vi "wfm_feature set_search_plot_pos.vi"(8 "error in (no error)":errorcluster, 10 "new search plot pos":cluster{"Array":cluster{"X":dbl, "Y":dbl}[]}, 11 "wfm_feature in":refnum<class "wfm_feature.lvclass">) -> (0 "error out":errorcluster, 3 "wfm_feature out":refnum<class "wfm_feature.lvclass">)   [LabVIEW 2018, in "wfm_feature.lvclass"]
uses:
  wfm_feature.lvclass
  wfm_feature.lvclass/wfm_feature.ctl
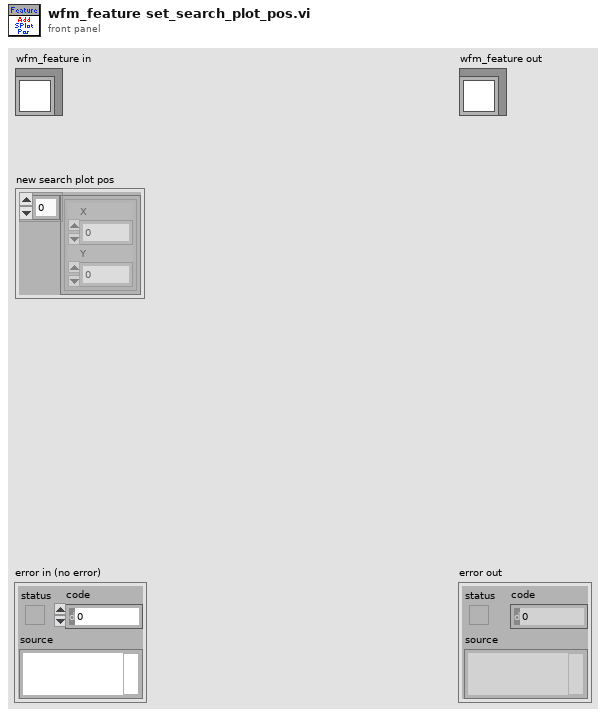
[diagram p1: front panel]
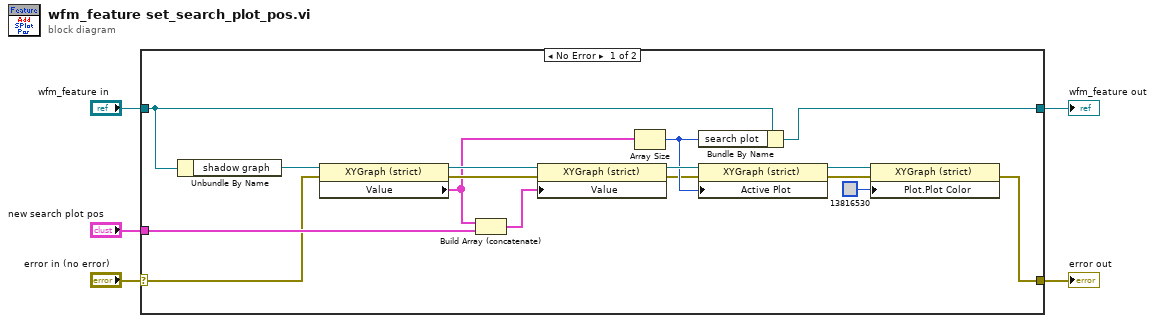
[diagram p0: block diagram]
diagram:
  n1 = case shown="No Error" "error in (no error)" {
    selector: "error in (no error)" -> [w14 w23]
    tunnel: [w6 w23] -> w4
    tunnel: [w15 w22] -> w2
    tunnel: "wfm_feature in" -> [w13 w22]
    tunnel: "new search plot pos" -> [w18 _]
    frame No Error {
      n2 = Unbundle By Name(w13) -> ("shadow graph"=w21:refnum<vi>)
      n3 = property class="XYGraph (strict)"(reference=w21, error in=w14) -> (reference out=w20:refnum<vi>, error out=w19:errorcluster, "Value"=w16:cluster{"Array":cluster{"X":dbl, "Y":dbl}[]}[])
      n4 = Build Array (concatenate)(w16, w18) -> (w17:cluster{"Array":cluster{"X":dbl, "Y":dbl}[]}[])
      n5 = property class="XYGraph (strict)"(reference=w20, error in=w19, "Value"=w17) -> (reference out=w12:refnum<vi>, error out=w10:errorcluster)
      n6 = Array Size(array=w16) -> (size(s)=w11:i32)
      n7 = Bundle By Name(cluster=w13, "search plot"=w11) -> (w15:refnum<class "wfm_feature.lvclass">)
      n8 = property class="XYGraph (strict)"(reference=w12, error in=w10, "Active Plot"=w11) -> (reference out=w9:refnum<vi>, error out=w8:errorcluster)
      n9 = property class="XYGraph (strict)"(reference=w9, error in=w8, "Plot.Plot Color"=u32 13816530) -> (error out=w6:errorcluster)  [unwired: 1 out]
    }
    frame Error {
    }
  }
  "error out" <- w4
  "wfm_feature out" <- w2
